vi "Haydonkerk14_step_motor.vi"(6 "F_Threshold":fxp<+,12,12>, 8 "dFmr":fxp<+/-,25,15>, 10 "omega":fxp<+/-,20,9>, 11 "Fmr":fxp<+/-,20,10>) -> (1 "vq_F":fxp<+/-,20,5> format="%.57g", 3 "vd_F":fxp<+/-,20,5>)   [LabVIEW 2014]
uses:
  <vilib>/rvi/FXPMathLib/FxpMul/XNode/nifxpmath_Multiplier.xnode
  <vilib>/rvi/FXPMathLib/FxpAdd/XNode/nifxpmath_Add.xnode
  <vilib>/rvi/FXPMathLib/sim/FxpSim.dll
panel:
  out "Lmdtau_mr/Km":fxp<+/-,30,15>
  out "-RKm/NrL":fxp<+/-,18,3>=-1.9615478515625
  out "tauR/Km":fxp<+/-,30,15>
  out "Kmw":fxp<+/-,25,10> format="%.50g"
  out "-NrLwtau/Km":fxp<+/-,28,9> format="%.54g"
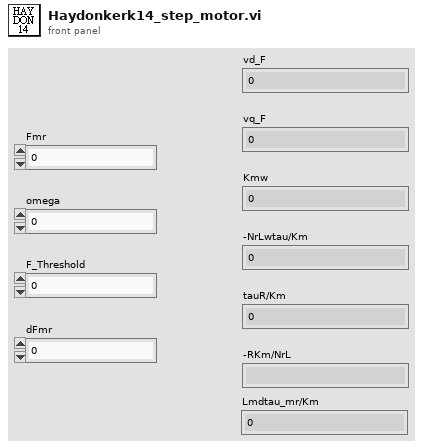
[diagram p1: front panel]
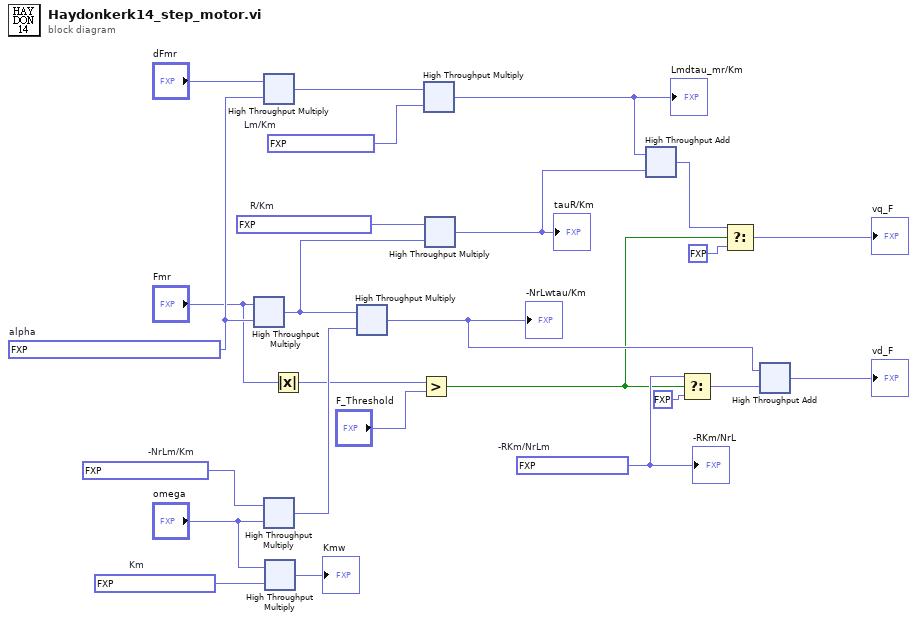
[diagram p0: block diagram]
diagram:
  w18 = fxp<+,23,7> 0.1177978515625  # Lm/Km
  w14 = fxp<+/-,20,4> -5.869476318359375  # -NrLm/Km
  w12 = fxp<+/-,18,3> -2.0596923828125  # -RKm/NrLm
  w21 = fxp<+,23,7> 83.73023986816406  # R/Km
  w9 = fxp<+,14,-2> 0.144866943359375  # Km
  w15 = fxp<+/-,28,0> 0.00038515403866767883  # alpha
  n1 = xnode ("High Throughput Multiply")("x"="Fmr", "y"=w15) -> ("x*y"=w10:fxp<+/-,28,9>)
  n2 = xnode ("High Throughput Multiply")("x"="dFmr", "y"=w15) -> ("x*y"=w11:fxp<+/-,28,9>)
  n3 = xnode ("High Throughput Multiply")("x"=w14, "y"="omega") -> ("x*y"=w13:fxp<+/-,28,9>)
  n4 = xnode ("High Throughput Multiply")("x"="omega", "y"=w9) -> ("x*y"=→"Kmw":fxp<+/-,22,7>)
  n5 = Absolute Value(x="Fmr") -> (abs(x)=w6:fxp<+,20,10>)
  n6 = xnode ("High Throughput Multiply")("x"=w10, "y"=w13) -> ("x*y"=w4:fxp<+/-,28,9>)
  "-NrLwtau/Km" <- w4
  n7 = Greater?(x=w6, y="F_Threshold") -> (0:w2:bool)
  n8 = xnode ("High Throughput Multiply")("x"=w11, "y"=w18) -> ("x*y"=w17:fxp<+/-,20,5>)
  "Lmdtau_mr/Km" <- w17
  n9 = xnode ("High Throughput Multiply")("x"=w21, "y"=w10) -> ("x*y"=w20:fxp<+/-,20,5>)
  "tauR/Km" <- w20
  n10 = xnode ("High Throughput Add")("x"=w17, "y"=w20) -> ("x+y"=w19:fxp<+/-,20,5>)
  n11 = Select(t=w12, s=w2, f=fxp<+/-,18,3> 0.0) -> (s? t:f=w3:fxp<+/-,18,3>)
  n12 = Select(t=w19, s=w2, f=fxp<+/-,20,5> 0.0) -> (s? t:f=→"vq_F":fxp<+/-,20,5>)
  n13 = xnode ("High Throughput Add")("x"=w4, "y"=w3) -> ("x+y"=→"vd_F":fxp<+/-,20,5>)
  "-RKm/NrL" <- w12
